vi "Message Callback.vi"(7 "Owner":refnum<class>, 11 "Message":refnum<class "Message.lvclass">) -> (0 "error out":errorcluster)   [LabVIEW 2020, in "LV Client.lvclass"]
uses:
  LV Client.lvclass
  LV Client.lvclass/LV Client.ctl
  <vilib>/IlluminatedG/lv-msg-simple/Stream-Simple-Msg/Message/Message.lvclass
  Common/Message ID.ctl
  Common/Common.lvlib
  cb1da58f-4d52-439a-a472-3e49e0b4ed0a.vi
  9bc2f38f-8094-4d0b-bada-c833bf8adefc.vi
  89d835f1-ac81-4984-9ff7-37f186ebb978.vi
  Common/Timer Init.ctl
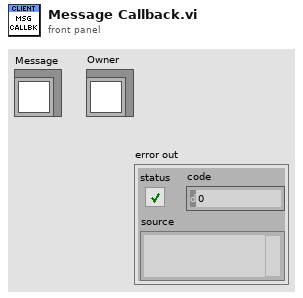
[diagram p1: front panel]
types:
  T1 = typedef "Common.lvlib/Message ID.ctl" = enum16{"Timer State", "Timer Value", "Timer Start", "Timer Pause", "Timer Reset", "Timer Init"}
  T2 = typedef "Common.lvlib/Timer Init.ctl" = cluster{"State":string, "Value":string}
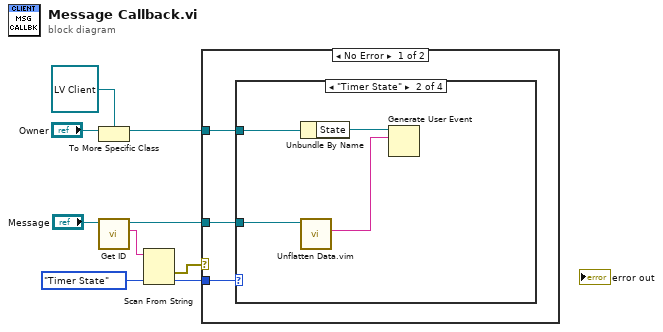
[diagram p0: block diagram]
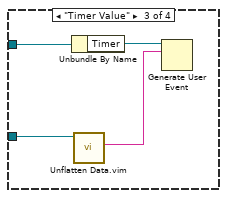
[diagram p3: hidden frame]
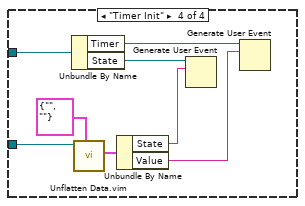
[diagram p4: hidden frame]
diagram:
  n1 = To More Specific Class(target class=refnum<class "LV Client.lvclass"> refnum ("LV Client.lvclass"), reference="Owner") -> (specific class reference=w2:refnum<class "LV Client.lvclass">)  [unwired: 1 in, 1 out]
  n2 = call <vilib>:"Get ID.vi"("Message in"="Message") -> ("ID"=w6:string, "Message out"=w1:refnum<class "Message.lvclass">)  [unwired: 8 in, 1 out]
  n3 = Scan From String(input string=w6, default 1=Message_ID."Timer State" ("Message ID")) -> (error out=w4:errorcluster, output 1=w3:T1)  [unwired: 3 in, 2 out]
  n4 = case shown="No Error" w4 {
    tunnel: w3 -> [w12 _]
    tunnel: w2 -> [w11 _]
    tunnel: w1 -> [w10 _]
    frame No Error {
      n5 = case shown="\"Timer State\"" w12 {
        tunnel: w11 -> [_ w16 w20 w28]
        tunnel: w10 -> [_ w14 w18 w26]
        frame Default {
        }
        frame "Timer State" {
          n6 = Unbundle By Name(w16) -> ("State"=w15:refnum<user-event>)
          n7 = call "Unflatten Data.vim"("Message in"=w14) -> ("Unflattened Data"=w13:string)  [unwired: 8 in, 2 out]
          n8 = Generate User Event(user event=w15, event data cluster=w13) -> ()  [unwired: 2 in, 2 out]
        }
        frame "Timer Value" {
          n9 = Unbundle By Name(w20) -> ("Timer"=w19:refnum<user-event>)
          n10 = call "Unflatten Data.vim"("Message in"=w18) -> ("Unflattened Data"=w17:string)  [unwired: 8 in, 2 out]
          n11 = Generate User Event(user event=w19, event data cluster=w17) -> ()  [unwired: 2 in, 2 out]
        }
        frame "Timer Init" {
          n12 = Unbundle By Name(w28) -> ("Timer"=w27:refnum<user-event>, "State"=w23:refnum<user-event>)
          n13 = call "Unflatten Data.vim"("Data Type (String)"=T2 {"State"="", "Value"=""} ("Timer Init"), "Message in"=w26) -> ("Unflattened Data"=w24:T2)  [unwired: 7 in, 2 out]
          n14 = Unbundle By Name(w24) -> ("State"=w22:string, "Value"=w21:string)
          n15 = Generate User Event(user event=w23, event data cluster=w22) -> ()  [unwired: 2 in, 2 out]
          n16 = Generate User Event(user event=w27, event data cluster=w21) -> ()  [unwired: 2 in, 2 out]
        }
      }
    }
    frame Error {
    }
  }
